vi "Process GD Info Cluster.vi"(8 "Sprachliste":string[][](array[string]), 11 "GD Info-Cluster in":T1) -> (2 "Störung":bool, 3 "String":string)   [LabVIEW 2020]
uses:
  GD Info Cluster.ctl
  LIN ErrorCluster.ctl
  SpanEinstellungen.lvlib
  Linearisierung v2.lvlib
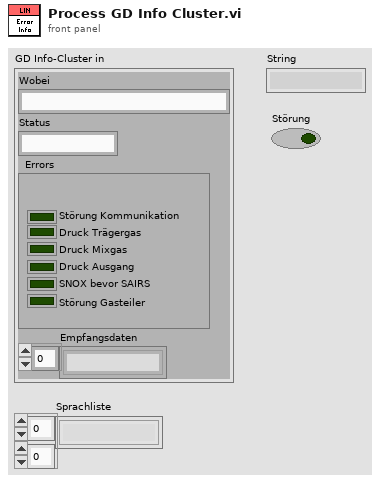
[diagram p1: front panel]
types:
  T1 = typedef "Linearisierung v2.lvlib/SpanEinstellungen.lvlib/GD Info Cluster.ctl" = cluster{"Wobei":string, "Status":string, "Errors":T2, "Empfangsdaten":string[]}
  T2 = typedef "Linearisierung v2.lvlib/LIN ErrorCluster.ctl" = cluster{"Störung Kommunikation":bool, "Pressure carrier gas":bool, "Pressure diluted gas":bool, "Outlet Pressure":bool, "SNOX before SAIR":bool, "Störung Gasteiler":bool}
  T3 = cluster{"Label.Text":string, "Störung Kommunikation":bool}[]
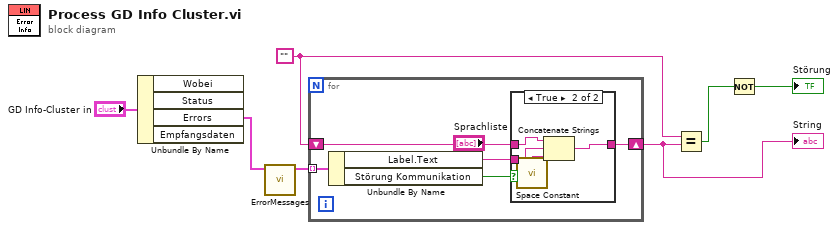
[diagram p0: block diagram]
diagram:
  w4 = ""
  n1 = Unbundle By Name("GD Info-Cluster in") -> ("Errors"=w1:T2)  [unwired: 3 out]
  n2 = call "ErrorMessages.vi"("Errors"=w1) -> ("Error Array"=w5:T3)  [unwired: 9 in, 1 out]
  n3 = for {
    tunnel: w5 -> [w12] mode=indexing
    shift-right: [w9] -> w7
    shift-left: w4 -> [w8]
    n4 = Unbundle By Name(w12) -> ("Label.Text"=w10:string, "Störung Kommunikation"=w11:bool)
    n5 = case shown="True" w11 {
      tunnel: w10 -> [_ w17]
      tunnel: [w13 w16] -> w9
      tunnel: w8 -> [w13 w14]
      frame False {
      }
      frame True {
        n6 = call <vilib>:"Space Constant.vi"() -> ("String"=w15:string)
        n7 = Concatenate Strings(w14, w17, w15) -> (w16:string)
      }
    }
  }
  "String" <- w7
  n8 = Equal?(x=w4, y=w7) -> (x = y?=w3:bool)
  n9 = Not(x=w3) -> (.not. x?=→"Störung":bool)
